vi "Agilis cfg Ch1Ax1Pos.vi"(8 "error in (no error)":errorcluster, 9 "Channel parsed command info":T1, 10 "Simulation":T2, 11 "input cluster":refnum<class "AgilisPiezoStage.lvclass">) -> (0 "error out":errorcluster, 1 "new commands":string, 3 "output cluster":refnum<class "AgilisPiezoStage.lvclass">)   [LabVIEW 2013, in "AgilisPiezoStage.lvclass"]
uses:
  AgilisPiezoStage.lvclass
  shared/OnOffTypeDef.ctl
  Shared/Device Driver/channel parsed cmd cluster.ctl
  AgilisPiezoStage.lvclass/AgilisPiezoStage.ctl
  C:/Program Files/Newport/Piezo Motion Control/Newport AG-UC2-UC8 Applet/Samples/LabVIEW 2009/AgilisCmdLib.dll
  Program Files/Newport/Piezo Motion Control/Newport AG-UC2-UC8 Applet/Samples/LabVIEW 2009/AgilisCmdLib.dll
  shared/CompressAndUpdate(Poly)/CompressAndUpdate(Numeric).vi
panel:
  out "errstring":string
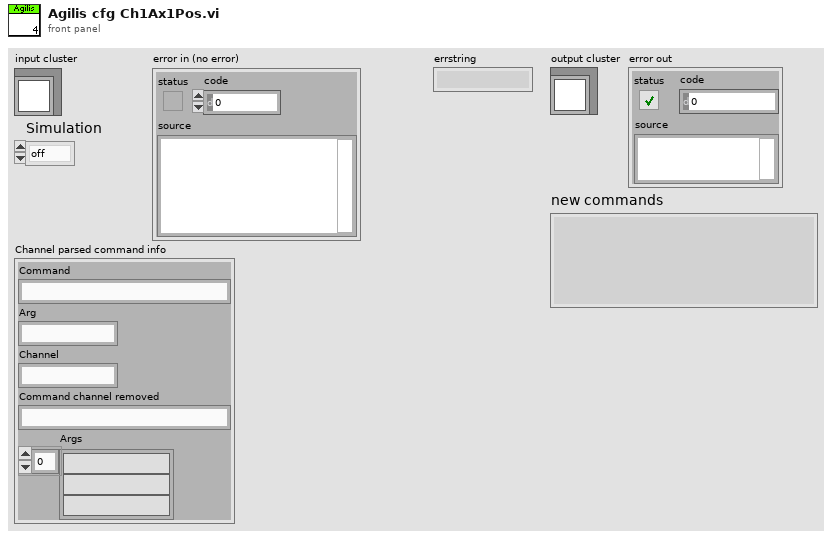
[diagram p1: front panel]
types:
  T1 = typedef "channel parsed cmd cluster.ctl" = cluster{"Command":string, "Arg":string, "Channel":string, "Command channel removed":string, "Args":string[]}
  T2 = typedef "OnOffTypeDef.ctl" = enum16{"off", "on"}
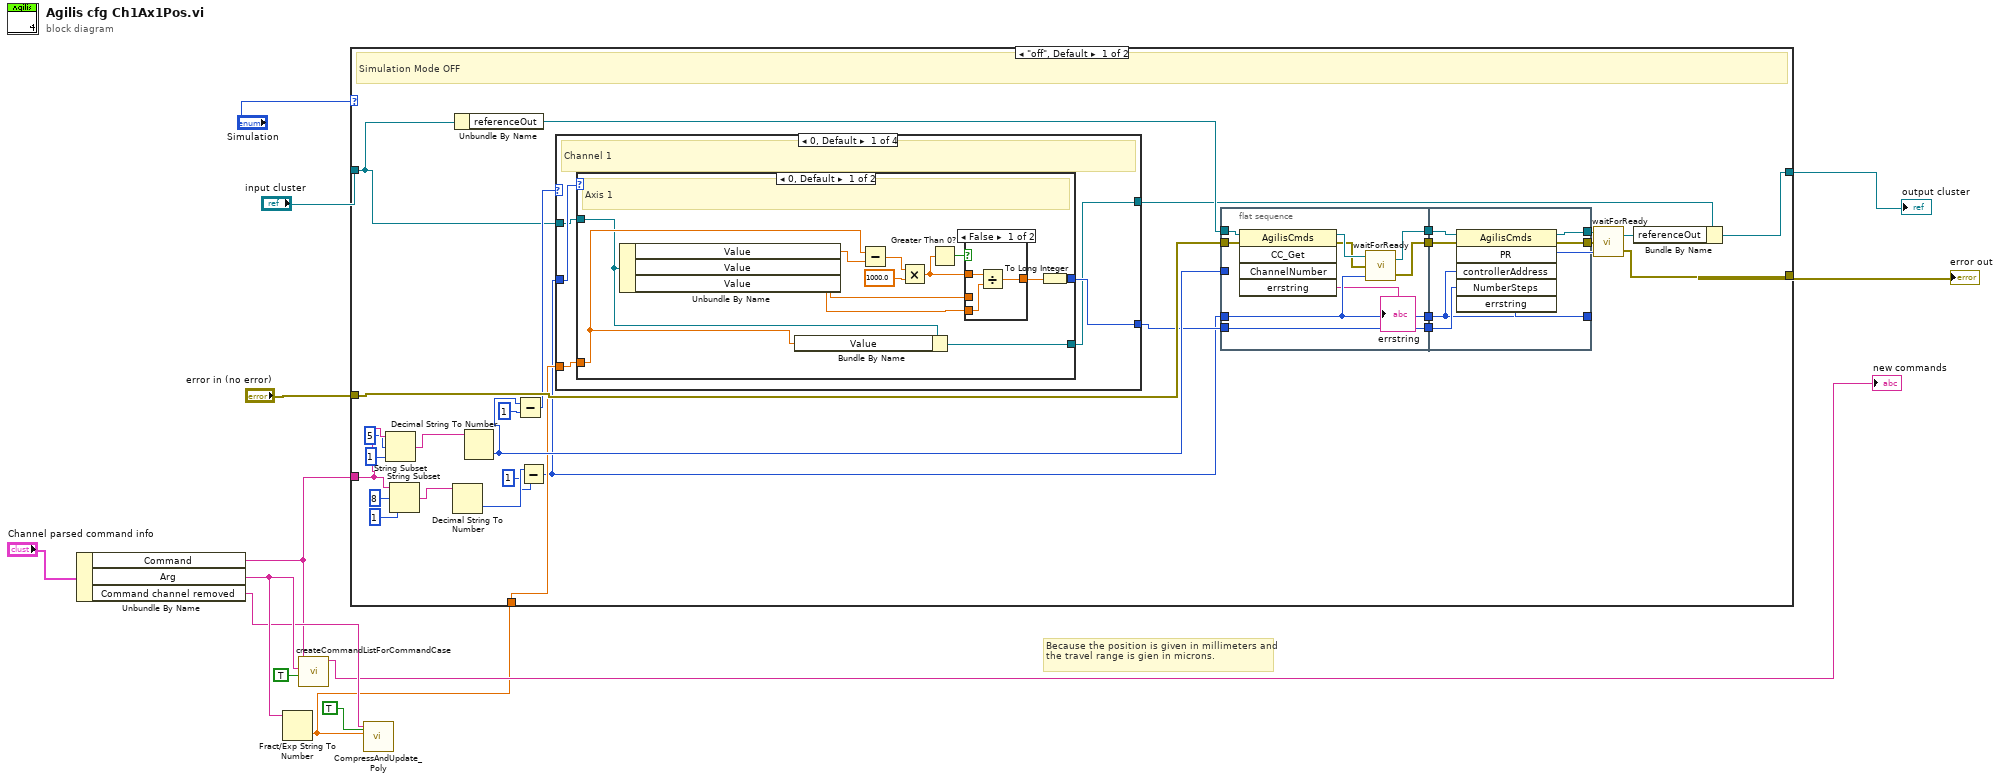
[diagram p0: block diagram]
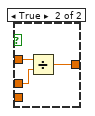
[diagram p2: hidden frame]
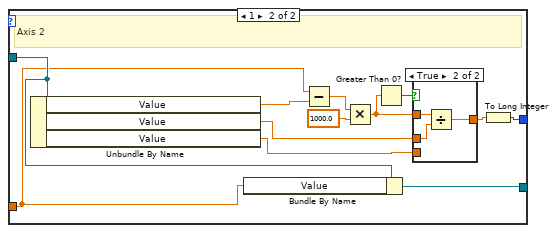
[diagram p3: hidden frame]
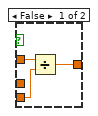
[diagram p4: hidden frame]
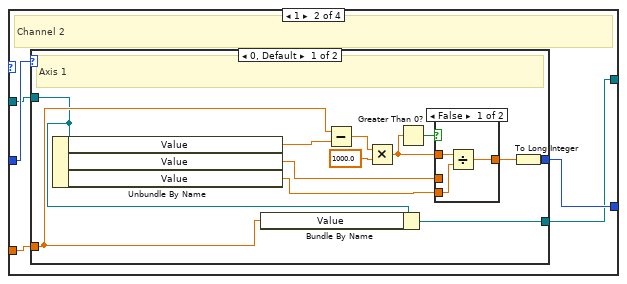
[diagram p5: hidden frame]
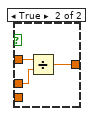
[diagram p6: hidden frame]
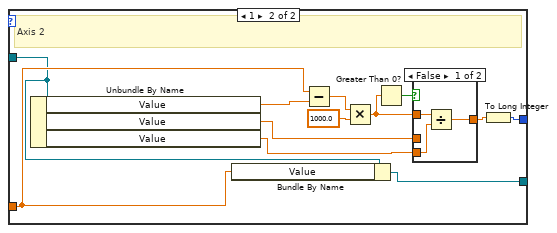
[diagram p7: hidden frame]
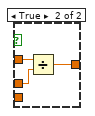
[diagram p8: hidden frame]
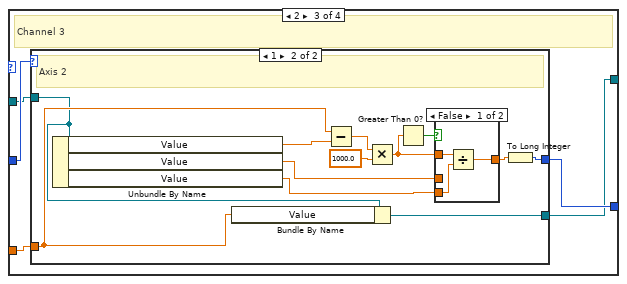
[diagram p9: hidden frame]
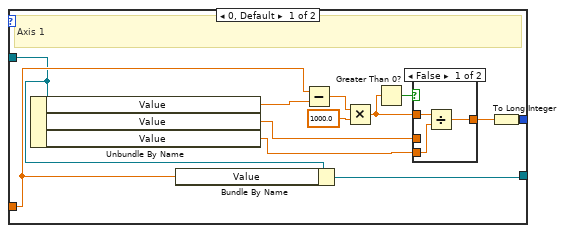
[diagram p10: hidden frame]
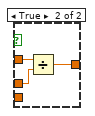
[diagram p11: hidden frame]
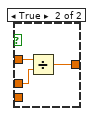
[diagram p12: hidden frame]
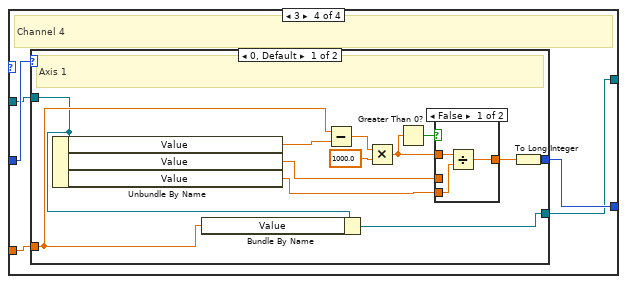
[diagram p13: hidden frame]
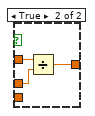
[diagram p14: hidden frame]
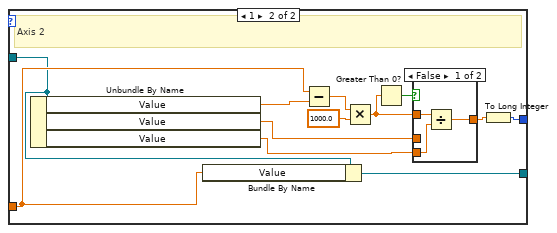
[diagram p15: hidden frame]
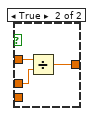
[diagram p16: hidden frame]
diagram:
  # "Because the position is given in millimeters and the travel range is gien in microns."
  n1 = Unbundle By Name("Channel parsed command info") -> ("Command"=w1:string, "Arg"=w10:string, "Command channel removed"=w9:string)
  n2 = Fract/Exp String To Number(string=w10) -> (number=w2:dbl)  [unwired: 3 in, 1 out]
  n3 = call "createCommandListForCommandCase.vi"("immediate Check (only once)"=TRUE, "setvalue"=w10, "command"=w1) -> ("new commands"=→"new commands":string)  [unwired: 8 in]
  n4 = case shown="\"off\", Default" "Simulation" {
    tunnel: [w25 w223] -> w5
    tunnel: "input cluster" -> [w27 w223]
    tunnel: "error in (no error)" -> [w41 w222]
    tunnel: [w39 w222] -> w4
    tunnel: w2 -> [w28 _]
    tunnel: w1 -> [w24 _]
    frame "off", Default {
      # "Simulation Mode OFF"
      n5 = String Subset(string=w24, offset (0)=5, length (rest)=1 ("length (rest)")) -> (substring=w37:string)
      n6 = String Subset(string=w24, offset (0)=8, length (rest)=1 ("length (rest)")) -> (substring=w34:string)
      n7 = Decimal String To Number(string=w34) -> (number=w30:i32)  [unwired: 2 in, 1 out]
      n8 = Unbundle By Name(w27) -> ("referenceOut"=w42:refnum<k24>)
      n9 = Decimal String To Number(string=w37) -> (number=w33:i32)  [unwired: 2 in, 1 out]
      n10 = Subtract(x=w33, y=1) -> (x-y=w31:i32)
      n11 = Subtract(x=w30, y=1) -> (x-y=w18:i32)
      n12 = case shown="0, Default" w31 {
        tunnel: w18 -> [w62 w103 w144 w185]
        tunnel: w28 -> [w61 w102 w143 w184]
        tunnel: w27 -> [w60 w101 w142 w183]
        tunnel: [w59 w100 w141 w182] -> w19
        tunnel: [w58 w99 w140 w181] -> w26
        frame 0, Default {
          # "Channel 1"
          n13 = case shown="0, Default" w62 {
            tunnel: w61 -> [w65 w82]
            tunnel: w60 -> [w63 w83]
            tunnel: [w66 w84] -> w59
            tunnel: [w64 w81] -> w58
            frame 0, Default {
              # "Axis 1"
              n14 = Unbundle By Name(w63) -> ("Value"=w69:dbl, "Value"=w68:dbl, "Value"=w67:dbl)
              n15 = Bundle By Name(cluster=w63, "Value"=w65) -> (w64:refnum<class "AgilisPiezoStage.lvclass">)
              n16 = Subtract(x=w65, y=w69) -> (x-y=w74:dbl)
              n17 = Multiply(x=w74, y=1000.0) -> (x*y=w71:dbl)
              n18 = Greater Than 0?(x=w71) -> (x > 0?=w72:bool)
              n19 = case shown="False" w72 {
                tunnel: w71 -> [w77 w80]
                tunnel: [w76 w79] -> w70
                tunnel: w68 -> [_ w78]
                tunnel: w67 -> [w75 _]
                frame False {
                  n20 = Divide(x=w77, y=w75) -> (x/y=w76:dbl)
                }
                frame True {
                  n21 = Divide(x=w80, y=w78) -> (x/y=w79:dbl)
                }
              }
              n22 = To Long Integer(number=w70) -> (32bit integer=w66:i32)
            }
            frame 1 {
              # "Axis 2"
              n23 = Unbundle By Name(w83) -> ("Value"=w87:dbl, "Value"=w86:dbl, "Value"=w85:dbl)
              n24 = Bundle By Name(cluster=w83, "Value"=w82) -> (w81:refnum<class "AgilisPiezoStage.lvclass">)
              n25 = Subtract(x=w82, y=w87) -> (x-y=w92:dbl)
              n26 = Multiply(x=w92, y=1000.0) -> (x*y=w89:dbl)
              n27 = Greater Than 0?(x=w89) -> (x > 0?=w90:bool)
              n28 = case shown="True" w90 {
                tunnel: w89 -> [w95 w98]
                tunnel: [w94 w97] -> w88
                tunnel: w86 -> [_ w96]
                tunnel: w85 -> [w93 _]
                frame False {
                  n29 = Divide(x=w95, y=w93) -> (x/y=w94:dbl)
                }
                frame True {
                  n30 = Divide(x=w98, y=w96) -> (x/y=w97:dbl)
                }
              }
              n31 = To Long Integer(number=w88) -> (32bit integer=w84:i32)
            }
          }
        }
        frame 1 {
          # "Channel 2"
          n32 = case shown="0, Default" w103 {
            tunnel: w102 -> [w106 w124]
            tunnel: w101 -> [w105 w123]
            tunnel: [w107 w125] -> w100
            tunnel: [w104 w122] -> w99
            frame 0, Default {
              # "Axis 1"
              n33 = Unbundle By Name(w105) -> ("Value"=w110:dbl, "Value"=w109:dbl, "Value"=w108:dbl)
              n34 = Bundle By Name(cluster=w105, "Value"=w106) -> (w104:refnum<class "AgilisPiezoStage.lvclass">)
              n35 = Subtract(x=w106, y=w110) -> (x-y=w115:dbl)
              n36 = Multiply(x=w115, y=1000.0) -> (x*y=w112:dbl)
              n37 = Greater Than 0?(x=w112) -> (x > 0?=w113:bool)
              n38 = case shown="False" w113 {
                tunnel: w112 -> [w118 w121]
                tunnel: [w117 w120] -> w111
                tunnel: w109 -> [_ w119]
                tunnel: w108 -> [w116 _]
                frame False {
                  n39 = Divide(x=w118, y=w116) -> (x/y=w117:dbl)
                }
                frame True {
                  n40 = Divide(x=w121, y=w119) -> (x/y=w120:dbl)
                }
              }
              n41 = To Long Integer(number=w111) -> (32bit integer=w107:i32)
            }
            frame 1 {
              # "Axis 2"
              n42 = Unbundle By Name(w123) -> ("Value"=w128:dbl, "Value"=w127:dbl, "Value"=w126:dbl)
              n43 = Bundle By Name(cluster=w123, "Value"=w124) -> (w122:refnum<class "AgilisPiezoStage.lvclass">)
              n44 = Subtract(x=w124, y=w128) -> (x-y=w133:dbl)
              n45 = Multiply(x=w133, y=1000.0) -> (x*y=w130:dbl)
              n46 = Greater Than 0?(x=w130) -> (x > 0?=w131:bool)
              n47 = case shown="False" w131 {
                tunnel: w130 -> [w136 w139]
                tunnel: [w135 w138] -> w129
                tunnel: w127 -> [_ w137]
                tunnel: w126 -> [w134 _]
                frame False {
                  n48 = Divide(x=w136, y=w134) -> (x/y=w135:dbl)
                }
                frame True {
                  n49 = Divide(x=w139, y=w137) -> (x/y=w138:dbl)
                }
              }
              n50 = To Long Integer(number=w129) -> (32bit integer=w125:i32)
            }
          }
        }
        frame 2 {
          # "Channel 3"
          n51 = case shown="1" w144 {
            tunnel: w143 -> [w147 w165]
            tunnel: w142 -> [w146 w164]
            tunnel: [w148 w166] -> w141
            tunnel: [w145 w163] -> w140
            frame 0, Default {
              # "Axis 1"
              n52 = Unbundle By Name(w146) -> ("Value"=w151:dbl, "Value"=w150:dbl, "Value"=w149:dbl)
              n53 = Bundle By Name(cluster=w146, "Value"=w147) -> (w145:refnum<class "AgilisPiezoStage.lvclass">)
              n54 = Subtract(x=w147, y=w151) -> (x-y=w156:dbl)
              n55 = Multiply(x=w156, y=1000.0) -> (x*y=w153:dbl)
              n56 = Greater Than 0?(x=w153) -> (x > 0?=w154:bool)
              n57 = case shown="False" w154 {
                tunnel: w153 -> [w159 w162]
                tunnel: [w158 w161] -> w152
                tunnel: w150 -> [_ w160]
                tunnel: w149 -> [w157 _]
                frame False {
                  n58 = Divide(x=w159, y=w157) -> (x/y=w158:dbl)
                }
                frame True {
                  n59 = Divide(x=w162, y=w160) -> (x/y=w161:dbl)
                }
              }
              n60 = To Long Integer(number=w152) -> (32bit integer=w148:i32)
            }
            frame 1 {
              # "Axis 2"
              n61 = Unbundle By Name(w164) -> ("Value"=w169:dbl, "Value"=w168:dbl, "Value"=w167:dbl)
              n62 = Bundle By Name(cluster=w164, "Value"=w165) -> (w163:refnum<class "AgilisPiezoStage.lvclass">)
              n63 = Subtract(x=w165, y=w169) -> (x-y=w174:dbl)
              n64 = Multiply(x=w174, y=1000.0) -> (x*y=w171:dbl)
              n65 = Greater Than 0?(x=w171) -> (x > 0?=w172:bool)
              n66 = case shown="False" w172 {
                tunnel: w171 -> [w177 w180]
                tunnel: [w176 w179] -> w170
                tunnel: w168 -> [_ w178]
                tunnel: w167 -> [w175 _]
                frame False {
                  n67 = Divide(x=w177, y=w175) -> (x/y=w176:dbl)
                }
                frame True {
                  n68 = Divide(x=w180, y=w178) -> (x/y=w179:dbl)
                }
              }
              n69 = To Long Integer(number=w170) -> (32bit integer=w166:i32)
            }
          }
        }
        frame 3 {
          # "Channel 4"
          n70 = case shown="0, Default" w185 {
            tunnel: w184 -> [w188 w206]
            tunnel: w183 -> [w187 w205]
            tunnel: [w189 w207] -> w182
            tunnel: [w186 w204] -> w181
            frame 0, Default {
              # "Axis 1"
              n71 = Unbundle By Name(w187) -> ("Value"=w192:dbl, "Value"=w191:dbl, "Value"=w190:dbl)
              n72 = Bundle By Name(cluster=w187, "Value"=w188) -> (w186:refnum<class "AgilisPiezoStage.lvclass">)
              n73 = Subtract(x=w188, y=w192) -> (x-y=w197:dbl)
              n74 = Multiply(x=w197, y=1000.0) -> (x*y=w194:dbl)
              n75 = Greater Than 0?(x=w194) -> (x > 0?=w195:bool)
              n76 = case shown="False" w195 {
                tunnel: w194 -> [w200 w203]
                tunnel: [w199 w202] -> w193
                tunnel: w191 -> [_ w201]
                tunnel: w190 -> [w198 _]
                frame False {
                  n77 = Divide(x=w200, y=w198) -> (x/y=w199:dbl)
                }
                frame True {
                  n78 = Divide(x=w203, y=w201) -> (x/y=w202:dbl)
                }
              }
              n79 = To Long Integer(number=w193) -> (32bit integer=w189:i32)
            }
            frame 1 {
              # "Axis 2"
              n80 = Unbundle By Name(w205) -> ("Value"=w210:dbl, "Value"=w209:dbl, "Value"=w208:dbl)
              n81 = Bundle By Name(cluster=w205, "Value"=w206) -> (w204:refnum<class "AgilisPiezoStage.lvclass">)
              n82 = Subtract(x=w206, y=w210) -> (x-y=w215:dbl)
              n83 = Multiply(x=w215, y=1000.0) -> (x*y=w212:dbl)
              n84 = Greater Than 0?(x=w212) -> (x > 0?=w213:bool)
              n85 = case shown="False" w213 {
                tunnel: w212 -> [w218 w221]
                tunnel: [w217 w220] -> w211
                tunnel: w209 -> [_ w219]
                tunnel: w208 -> [w216 _]
                frame False {
                  n86 = Divide(x=w218, y=w216) -> (x/y=w217:dbl)
                }
                frame True {
                  n87 = Divide(x=w221, y=w219) -> (x/y=w220:dbl)
                }
              }
              n88 = To Long Integer(number=w211) -> (32bit integer=w207:i32)
            }
          }
        }
      }
      n89 = flat-sequence {
        tunnel: w42 -> [w51]
        tunnel: w41 -> [w50]
        tunnel: w33 -> [_]
        tunnel: [w45] -> w22
        tunnel: [w44] -> w21
        tunnel: [w49] -> w20
        tunnel: w19 -> [w49]
        tunnel: w18 -> [w48]
        tunnel: [w48] -> w17
        tunnel: [w53] -> w15
        tunnel: [w52] -> w16
        tunnel: w22 -> [w55]
        tunnel: w21 -> [w54]
        tunnel: w20 -> [w57]
        tunnel: w17 -> [w56]
        tunnel: [w56] -> w14
        frame #0 {
          n90 = invoke class="AgilisCmds" method="CC_Get"(reference=w51, error in=w50) -> (reference out=w47:refnum<k24>, error out=w46:errorcluster, "errstring"=→"errstring":string)  [unwired: 3 in, 2 out]
          n91 = call "waitForReady.vi"("axis"=w48, "errorIn"=w46, "referenceIn"=w47) -> ("errorOut"=w44:errorcluster, "referenceOut"=w45:refnum<k24>)
        }
        frame #1 {
          n92 = invoke class="AgilisCmds" method="PR"(reference=w55, error in=w54, "controllerAddress"=w56, "NumberSteps"=w57) -> (reference out=w52:refnum<k24>, error out=w53:errorcluster)  [unwired: 2 in, 4 out]
        }
      }
      n93 = call "waitForReady.vi"("axis"=w14, "errorIn"=w15, "referenceIn"=w16) -> ("errorOut"=w39:errorcluster, "referenceOut"=w40:refnum<k24>)
      n94 = Bundle By Name(cluster=w26, "referenceOut"=w40) -> (w25:refnum<class "AgilisPiezoStage.lvclass">)
    }
    frame "on" {
      # "Simulation Mode ON"
    }
  }
  "output cluster" <- w5
  "error out" <- w4
  n95 = call-poly "CompressAndUpdate_Poly.vi"("force CVT update (false)"=TRUE ("force CVT update"), "Numeric"=w2, "command or variable name"=w9) -> ()  [unwired: 8 in, 1 out]
